vi "MarbleDispenserMk5.vi"   [LabVIEW 2016]
uses:
  <vilib>/NXT/Block Support/NXT_InputPort.ctl
  <vilib>/NXT/Block Support/NXT_OutputPort.ctl
  <vilib>/NXT/Dual Mode Library/Sensors/EV3_Color_Reflect.vi
  <vilib>/NXT/Dual Mode Library/Sensors/Touch_Released.vi
  <vilib>/NXT/NXTIO Xnodes/NXTIONodeSubVIs/NXTStopMotors.vi
  <vilib>/NXT/NXTIO Xnodes/NXTIONodeSubVIs/NXTMoveMotors.vi
  <vilib>/NXT/NXTIO Xnodes/NXTIONodeSubVIs/NXTMotorRunDistance.vi
  <vilib>/NXT/Dual Mode Library/Waits/Wait_Num.vi
  <vilib>/NXT/Dual Mode Library/Sensors/Touch_Pressed.vi
  <vilib>/NXT/Dual Mode Library/Sensors/EV3_Color_Color.vi
  <vilib>/NXT/Subs/LVHSConnector.ctl
  <vilib>/NXT/NXTIO Xnodes/AddressXNode/NXTIOAddress.xnode
  <vilib>/NXT/NXTIO Xnodes/NXTIOXNode/NXTIO.xnode
  <vilib>/NXT/LegoClasses/BrickReference/BrickReference.lvclass
types:
  T1 = typedef "NXT_InputPort.ctl" = u32
  T2 = typedef "NXT_OutputPort.ctl" = u8
  T3 = typedef "LVHSConnector.ctl" = refnum<class "BrickReference.lvclass">
  T4 = typedef "ColorSensorColors.ctl" = enum16{"No Color", "Black", "Blue", "Green", "Yellow", "Red", "White", "Brown"}
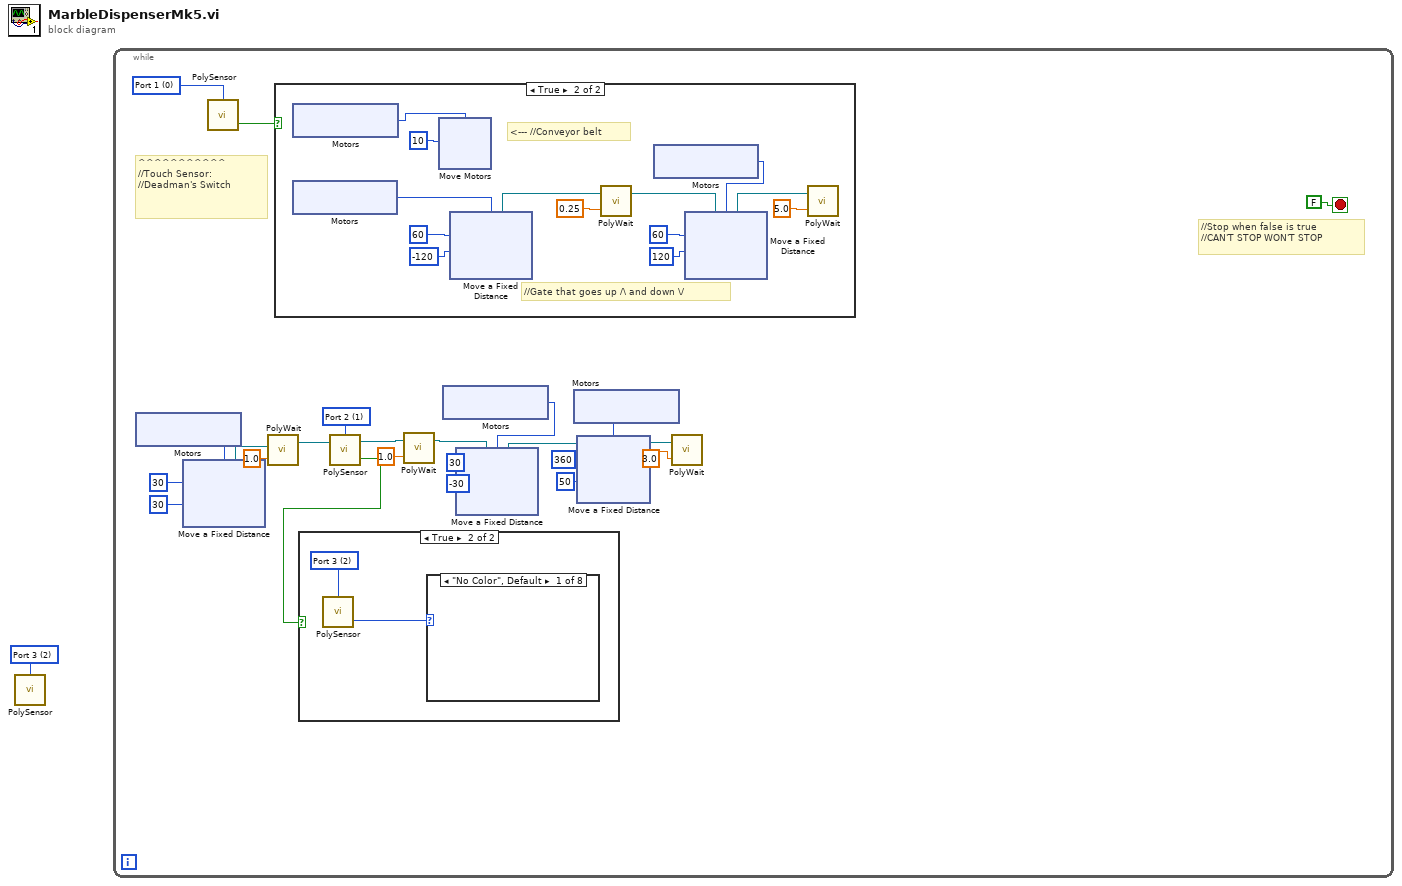
[diagram p0: block diagram]
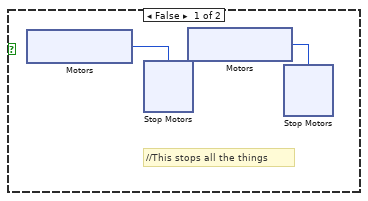
[diagram p10: hidden frame]
diagram:
  w1 = T1 2 items=["Port 1", "Port 2", "Port 3", "Port 4"] ("Port (Port 1)")
  n1 = call-poly <vilib>:"PolySensor.vi"("Port (Port 1)"=w1) -> ()  [unwired: 2 in, 2 out]
  n2 = while {
    stop <- FALSE stop-if-true
    w11 = T1 1 items=["Port 1", "Port 2", "Port 3", "Port 4"] ("Port (Port 1)")
    w24 = T1 0 items=["Port 1", "Port 2", "Port 3", "Port 4"] ("Port (Port 1)")
    # "//Stop when false is true\n//CAN'T STOP WON'T STOP"
    # "^^^^^^^^^^^\n//Touch Sensor:\n//Deadman's Switch"
    n3 = xnode "Motors"() -> ("Motor"=w17:T2)
    n4 = xnode "Move a Fixed Distance"("Speed 1"=30, "Distance 1"=30, "Motors"=w17) -> ("NXT/EV3"=w20:T3)  [unwired: 1 in]
    n5 = call-poly <vilib>:"PolySensor.vi"("Port (Port 1)"=w24) -> ("Yes / No"=w22:bool)  [unwired: 2 in, 1 out]
    n6 = call-poly <vilib>:"PolyWait.vi"("Time (1 sec)"=1.0, "NXT/EV3"=w20) -> ("NXT/EV3"=w12:T3)  [unwired: 2 in]
    n7 = case shown="True" w22 {
      frame False {
        # "//This stops all the things"
        n8 = xnode "Motors"() -> ("Motor"=w61:T2)
        n9 = xnode "Stop Motors"("Motors"=w61) -> ()  [unwired: 1 in, 1 out]
        n10 = xnode "Motors"() -> ("Motor"=w60:T2)
        n11 = xnode "Stop Motors"("Motors"=w60) -> ()  [unwired: 1 in, 1 out]
      }
      frame True {
        # "//Gate that goes up /\\ and down \\/"
        # "<--- //Conveyor belt"
        n12 = xnode "Motors"() -> ("Motor"=w86:T2)
        n13 = xnode "Motors"() -> ("Motor"=w80:T2)
        n14 = xnode "Move Motors"("Power/Speed 1"=10, "Motors"=w86) -> ()  [unwired: 1 in, 1 out]
        n15 = xnode "Move a Fixed Distance"("Speed 1"=-120, "Distance 1"=60, "Motors"=w80) -> ("NXT/EV3"=w83:T3)  [unwired: 1 in]
        n16 = call-poly <vilib>:"PolyWait.vi"("Time (1 sec)"=0.25, "NXT/EV3"=w83) -> ("NXT/EV3"=w75:T3)  [unwired: 2 in]
        n17 = xnode "Motors"() -> ("Motor"=w74:T2)
        n18 = xnode "Move a Fixed Distance"("Speed 1"=120, "Distance 1"=60, "Motors"=w74, "NXT/EV3"=w75) -> ("NXT/EV3"=w78:T3)
        n19 = call-poly <vilib>:"PolyWait.vi"("Time (1 sec)"=5.0, "NXT/EV3"=w78) -> ()  [unwired: 2 in, 1 out]
      }
    }
    n20 = call-poly <vilib>:"PolySensor.vi"("NXT/EV3"=w12, "Port (Port 1)"=w11) -> ("Yes / No"=w10:bool, "NXT/EV3"=w9:T3)  [unwired: 1 in]
    n21 = case shown="True" w10 {
      frame False {
      }
      frame True {
        w36 = T1 2 items=["Port 1", "Port 2", "Port 3", "Port 4"] ("Port (Port 1)")
        n22 = call-poly <vilib>:"PolySensor.vi"("Port (Port 1)"=w36) -> ("Detected Color"=w37:T4)  [unwired: 2 in, 1 out]
        n23 = case shown="\"No Color\", Default" w37 {
          frame "No Color", Default {
          }
          frame "Black" {
          }
          frame "Blue" {
          }
          frame "Green" {
          }
          frame "Yellow" {
          }
          frame "Red" {
          }
          frame "White" {
          }
          frame "Brown" {
          }
        }
      }
    }
    n24 = call-poly <vilib>:"PolyWait.vi"("Time (1 sec)"=sgl 1.0, "NXT/EV3"=w9) -> ("NXT/EV3"=w8:T3)  [unwired: 2 in]
    n25 = xnode "Motors"() -> ("Motor"=w13:T2)
    n26 = xnode "Move a Fixed Distance"("Speed 1"=-30, "Distance 1"=30, "Motors"=w13, "NXT/EV3"=w8) -> ("NXT/EV3"=w6:T3)
    n27 = xnode "Motors"() -> ("Motor"=w4:T2)
    n28 = xnode "Move a Fixed Distance"("Speed 1"=i8 50, "Distance 1"=360, "Motors"=w4, "NXT/EV3"=w6) -> ("NXT/EV3"=w5:T3)
    n29 = call-poly <vilib>:"PolyWait.vi"("Time (1 sec)"=3.0, "NXT/EV3"=w5) -> ()  [unwired: 2 in, 1 out]
  }
